vi "Get Top Node.vi"(8 "error in (no error)":errorcluster) -> (0 "error out":errorcluster, 2 "top node name":string, 3 "top node ref":refnum<vi>)   [LabVIEW 2014, in "lvprj2html.lvlib"]
uses:
  lvprj2html.lvlib
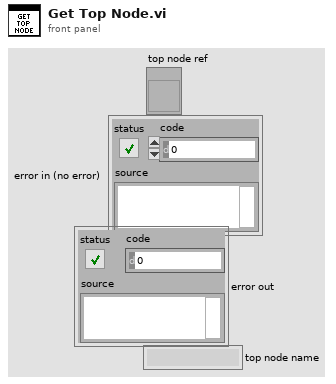
[diagram p1: front panel]
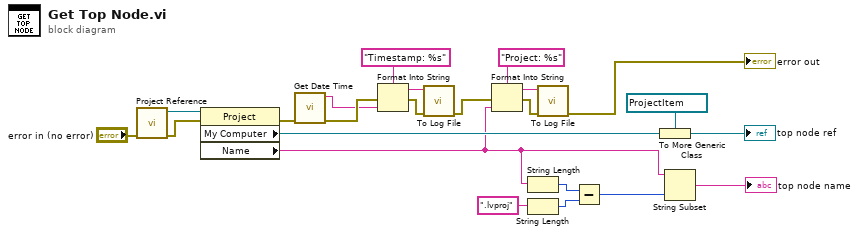
[diagram p0: block diagram]
diagram:
  n1 = call "Project Reference.vi"("error in (no error)"="error in (no error)") -> ("error out"=w18:errorcluster, "prj ref"=w20:refnum<vi>)  [unwired: 9 in]
  n2 = property class="Project"(reference=w20, error in=w18) -> (error out=w13:errorcluster, "My Computer"=w23:refnum<vi>, "Name"=w2:string)  [unwired: 1 out]
  n3 = call "Get Date Time.vi"("error in"=w13) -> ("error out"=w8:errorcluster, "date time"=w7:string)  [unwired: 9 in]
  n4 = Format Into String(format string="Timestamp: %s", error in=w8, w7) -> (resulting string=w10:string, error out=w11:errorcluster)  [unwired: 1 in]
  n5 = call "To Log File.vi"("error in (no error)"=w11, "string"=w10) -> ("error out"=w9:errorcluster)  [unwired: 9 in]
  n6 = Format Into String(format string="Project: %s", error in=w9, w2) -> (resulting string=w17:string, error out=w16:errorcluster)  [unwired: 1 in]
  n7 = String Length(string=w2) -> (length=w6:i32)
  n8 = String Length(string=".lvproj") -> (length=w5:i32)
  n9 = call "To Log File.vi"("error in (no error)"=w16, "string"=w17) -> ("error out"=→"error out":errorcluster)  [unwired: 9 in]
  n10 = Subtract(x=w6, y=w5) -> (x-y=w3:i32)
  n11 = To More Generic Class(target class=refnum<vi> refnum ("TargetItem in"), reference=w23) -> (generic class reference=→"top node ref":refnum<vi>)
  n12 = String Subset(string=w2, length (rest)=w3) -> (substring=→"top node name":string)  [unwired: 1 in]
